vi "Initialize.vi"(8 "error in (no error)":errorcluster, 9 "Reset (True)":bool=TRUE, 10 "ID Query (True)":bool=TRUE, 11 "VISA resource name":refnum<visa-resource-name>) -> (0 "error out":errorcluster, 2 "IDN":string, 3 "VISA resource name out":refnum<visa-resource-name>)   [LabVIEW 2020, in "HandsOnPi2040.lvlib"]
doc: "Establishes communication with the instrument and optionally performs an instrument identification query and/or an instrument reset. It also places the instrument in a default state needed for other instrument driver operations. Therefore, call this VI before calling other instrument driver VIs for this instrument. Generally, you need to call the <b>Initialize</b> VI only once at the beginning of an application."
uses:
  <instrlib>/HandsOnPi2040/HandsOnPi2040.lvlib
panel:
  # "Input"
  # "Output"
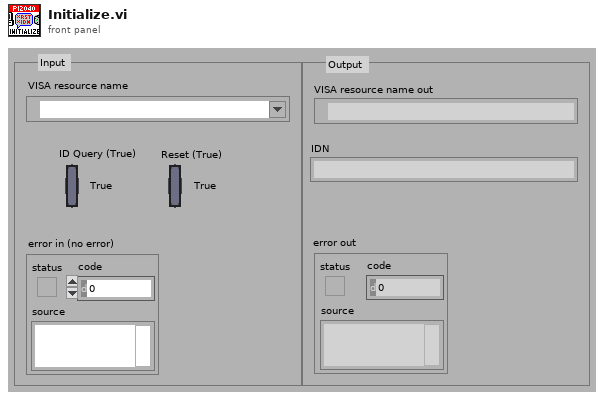
[diagram p1: front panel]
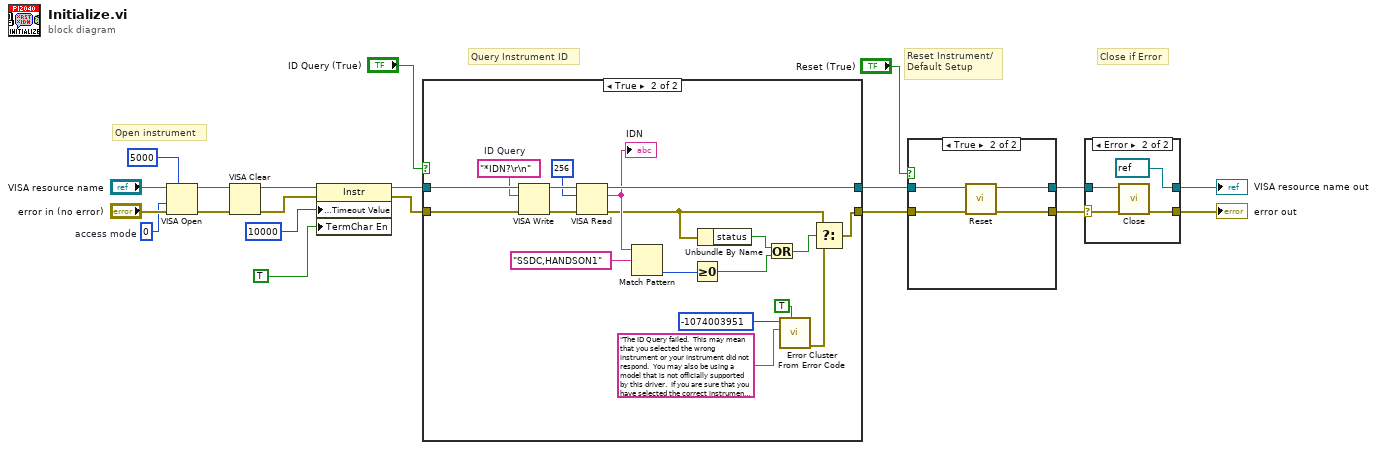
[diagram p0: block diagram]
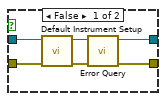
[diagram p3: hidden frame]
diagram:
  w11 = u32 0  # access mode
  # "Close if Error"
  # "Query Instrument ID"
  # "Reset Instrument/\nDefault Setup"
  # "Open instrument"
  n1 = VISA Open(timeout (0)=u32 5000 ("VISA Open timeout (0)"), access mode=w11, error in (no error)="error in (no error)", VISA resource name="VISA resource name") -> (VISA resource name=w10:refnum<visa-resource-name>, error out=w9:errorcluster)  [unwired: 1 in]
  n2 = VISA Clear(VISA resource name=w10, error in (no error)=w9) -> (VISA resource name out=w8:refnum<visa-resource-name>, error out=w7:errorcluster)
  n3 = property class="Instr"(reference=w8, error in=w7, "General Settings:Timeout Value"=u32 10000, "TermChar En"=TRUE ("Message Based Settings:Termination Character Enable")) -> (reference out=w13:refnum<visa-resource-name>, error out=w12:errorcluster)
  n4 = case shown="True" "ID Query (True)" {
    tunnel: [w21 w41] -> w19
    tunnel: [w22 w38] -> w20
    tunnel: w13 -> [w22 w39]
    tunnel: w12 -> [w21 w40]
    frame False {
    }
    frame True {
      w32 = "*IDN?\r\n"  # ID Query
      n5 = VISA Write(VISA resource name=w39, write buffer=w32, error in (no error)=w40) -> (VISA resource name out=w36:refnum<visa-resource-name>, error out=w35:errorcluster)  [unwired: 1 out]
      n6 = VISA Read(VISA resource name=w36, byte count=u32 256, error in (no error)=w35) -> (VISA resource name out=w38:refnum<visa-resource-name>, read buffer=w37:string, error out=w26:errorcluster)  [unwired: 1 out]
      "IDN" <- w37
      n7 = Match Pattern(string=w37, regular expression="SSDC,HANDSON1") -> (offset past match=w27:i32)  [unwired: 1 in, 3 out]
      n8 = Greater Or Equal To 0?(x=w27) -> (x >= 0?=w24:bool)
      n9 = Unbundle By Name(w26) -> ("status"=w25:bool)
      n10 = Or(x=w25, y=w24) -> (x .or. y?=w23:bool)
      n11 = call <vilib>:"Error Cluster From Error Code.vi"("show call chain? (False)"=TRUE, "error message (\"\")"="The ID Query failed.  This may mean that you selected the wrong instrument or your instrument did not respond.  You may also be using a model that is not officially supported by this driver.  If you are sure that you have selected the correct instrument and it is responding, try disabling the ID Query." ("Source (VI Name)"), "error code (0)"=-1074003951 ("Code")) -> ("error out"=w31:errorcluster)  [unwired: 6 in]
      n12 = Select(t=w26, s=w23, f=w31) -> (s? t:f=w41:errorcluster)
    }
  }
  n13 = case shown="True" "Reset (True)" {
    tunnel: w19 -> [w46 w48]
    tunnel: [w43 w51] -> w3
    tunnel: w20 -> [w47 w49]
    tunnel: [w44 w50] -> w4
    frame False {
      n14 = call <instrlib>:"Default Instrument Setup.vi"("error in (no error)"=w46, "VISA resource name"=w47) -> ("error out"=w42:errorcluster, "VISA resource name out"=w45:refnum<visa-resource-name>)  [unwired: 8 in]
      n15 = call <instrlib>:"Error Query.vi"("error in (no error)"=w42, "VISA resource name"=w45) -> ("error out"=w43:errorcluster, "VISA resource name out"=w44:refnum<visa-resource-name>)  [unwired: 6 in, 2 out]
    }
    frame True {
      n16 = call <instrlib>:"Reset.vi"("error in (no error)"=w48, "VISA resource name"=w49) -> ("error out"=w51:errorcluster, "VISA resource name out"=w50:refnum<visa-resource-name>)  [unwired: 8 in]
    }
  }
  n17 = case shown="Error" w3 {
    selector: w3 -> [w52 w55]
    tunnel: w4 -> [w53 w56]
    tunnel: [w53 refnum<visa-resource-name> refnum ("VISA resource name out")] -> w6
    tunnel: [w52 w57] -> w5
    frame No Error {
    }
    frame Error {
      n18 = call <instrlib>:"Close.vi"("error in (no error)"=w55, "VISA resource name"=w56) -> ("error out"=w57:errorcluster)  [unwired: 9 in]
    }
  }
  "VISA resource name out" <- w6
  "error out" <- w5
